vi "Write Engine Setting.vi"(8 "error in (no error)":errorcluster, 10 "Engine Setting":T1={"Enabled"=TRUE, "IP Address"="127.0.0.1", "Port"=3331, "Description"="Type = Class \n", "Type"="none", "Version"="1.0.0.0"}, 11 "Engine configuration in":refnum<class "Engine configuration.lvclass">) -> (0 "error out":errorcluster, 3 "Engine configuration out":refnum<class "Engine configuration.lvclass">)   [LabVIEW 2025, in "Abstract Engine.lvlib" / "Engine configuration.lvclass"]
uses:
  Engine configuration.lvclass
  Engine Setting.ctl
  Engine configuration.lvclass/Engine configuration.ctl
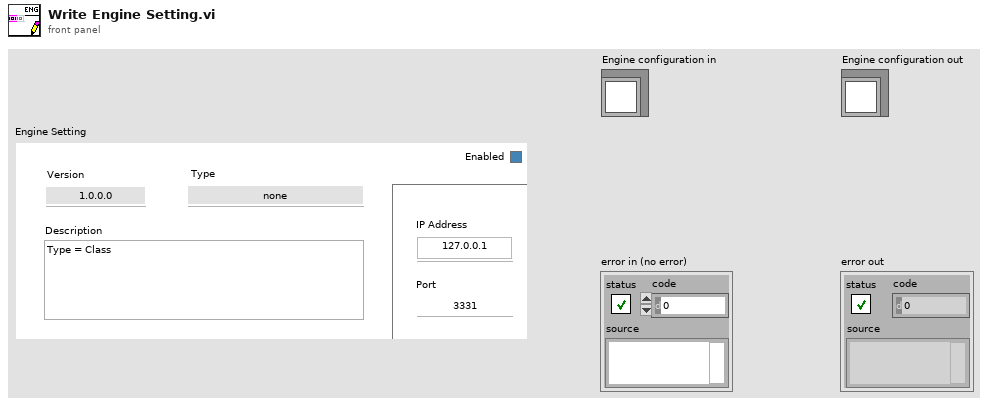
[diagram p1: front panel]
types:
  T1 = typedef "Abstract Engine.lvlib/Engine configuration.lvclass/Engine Setting.ctl" = cluster{"Enabled":bool, "IP Address":string, "Port":i32, "Description":string, "Type":string, "Version":string}
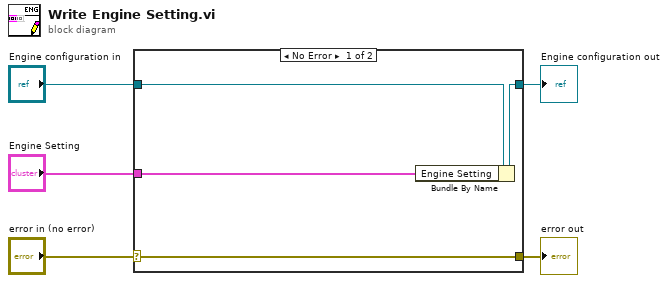
[diagram p0: block diagram]
diagram:
  n1 = case shown="No Error" "error in (no error)" {
    selector: "error in (no error)" -> [w9 w10]
    tunnel: [w9 w10] -> w4
    tunnel: [w7 w11] -> w2
    tunnel: "Engine configuration in" -> [w8 w11]
    tunnel: "Engine Setting" -> [w6 _]
    frame No Error {
      n2 = Bundle By Name(cluster=w8, "Engine Setting"=w6) -> (w7:refnum<class "Engine configuration.lvclass">)
    }
    frame Error {
    }
  }
  "error out" <- w4
  "Engine configuration out" <- w2
